vi "Get DateTime String.vi"() -> (1 "Time string":string, 3 "date/time string":string)   [LabVIEW 2013]
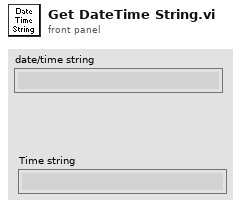
[diagram p1: front panel]
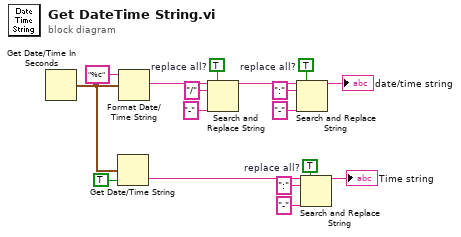
[diagram p0: block diagram]
diagram:
  w2 = TRUE  # replace all?
  w10 = TRUE  # replace all?
  w16 = TRUE  # replace all?
  n1 = Get Date/Time In Seconds() -> (seconds since 1Jan1904=w7:timestamp)
  n2 = Get Date/Time String(seconds (now)=w7, want seconds? (F)=TRUE) -> (time string=w1:string)  [unwired: 1 in, 1 out]
  n3 = Format Date/Time String(time format string (%c)="%c", seconds (now)=w7) -> (date/time string=w9:string)  [unwired: 1 in]
  n4 = Search and Replace String(replace all?=w10, input string=w9, search string="/", replace string="-" ("replace string (\"\")")) -> (result string=w8:string)  [unwired: 4 in, 3 out]
  n5 = Search and Replace String(replace all?=w16, input string=w8, search string=":", replace string="-" ("replace string (\"\")")) -> (result string=→"date/time string":string)  [unwired: 4 in, 3 out]
  n6 = Search and Replace String(replace all?=w2, input string=w1, search string=":", replace string="-" ("replace string (\"\")")) -> (result string=→"Time string":string)  [unwired: 4 in, 3 out]
